vi "Verify Row [  ].vi"(0 "Table size":cluster{"# Column":u16, "# Row":u16}, 7 "Row  [ ] IN":T1) -> (4 "Create Table?":bool, 8 "Row  [ ] OUT":T1)   [LabVIEW 2019]
doc: "Developed by Jean-Marc Simard\nCopyright © 2012, Exaprom Inc.\nAll rights reserved.\nLicense: BSD\n\nWith iTextSharp 4.1.6 (http://itextsharp.sourceforge.net)\nunder Mozilla Public License Version 1.1\n(http://www.mozilla.org/MPL/MPL-1.1.html)"
uses:
  <userlib>/Exaprom PDF/Controls/Table Controls/Table Appearance and Font Row [ ].ctl
  <userlib>/Exaprom PDF/Controls/Table Controls/One Row Appearance.ctl
  <userlib>/Exaprom PDF/Controls/Table Controls/Row from to.ctl
  <userlib>/Exaprom PDF/Controls/Table Controls/Cell, Alignment, LS and Font - hide Vmerge.ctl
  <userlib>/Exaprom PDF/Controls/Table Controls/Cell Type, Alignment and LS.ctl
  <userlib>/Exaprom PDF/Controls/Table Controls/Cell Alignment 20px.ctl
  <userlib>/Exaprom PDF/Controls/Table Controls/Text vertical arrangement.ctl
  <userlib>/Exaprom PDF/Controls/Text Controls/Line spacing.ctl
  <userlib>/Exaprom PDF/Controls/Table Controls/Cell Appearance.ctl
  <userlib>/Exaprom PDF/Controls/Table Controls/Cell Border 20 px.ctl
  <userlib>/Exaprom PDF/Controls/Table Controls/Merge Horizontal.ctl
  <userlib>/Exaprom PDF/Controls/Table Controls/Merge Vertical.ctl
  <userlib>/Exaprom PDF/Controls/Font Controls/Font complete cluster.ctl
  <userlib>/Exaprom PDF/Controls/Font Controls/Font size.ctl
  <userlib>/Exaprom PDF/Controls/Font Controls/Font color.ctl
  <userlib>/Exaprom PDF/Controls/Font Controls/Type and encoding.ctl
  <userlib>/Exaprom PDF/Controls/Text Controls/Unicode/Type and run direction.ctl
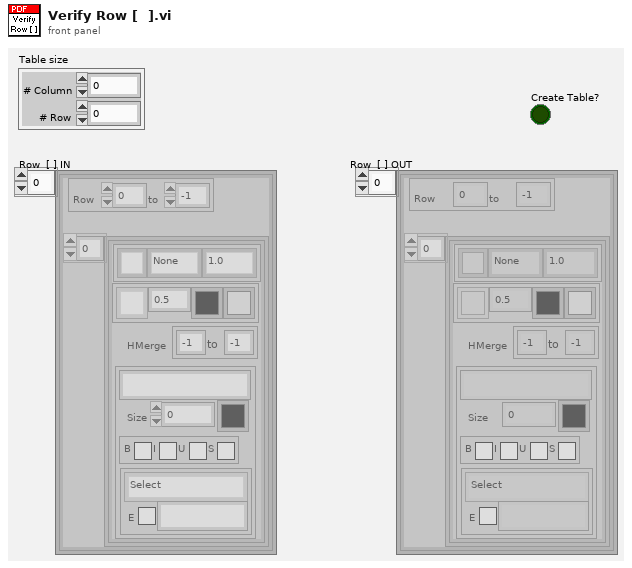
[diagram p1: front panel]
types:
  T1 = typedef "Table Appearance and Font Row [ ].ctl" = T2[]
  T2 = typedef "One Row Appearance.ctl" = cluster{"Row":T3, "Cell [ ]":T4[]}
  T3 = typedef "Row from to.ctl" = cluster{"From #":i16, "to #":i16}
  T4 = typedef "Cell, Alignment, LS and Font - hide Vmerge.ctl" = cluster{"Text":T5, "Cell Appearance":T9, "HMerge":T11, "VMerge":T12, "Font":T13}
  T5 = typedef "Cell Type, Alignment and LS.ctl" = cluster{"Cell Alignment":T6, "Text rotation":T7, "Line spacing":T8}
  T6 = typedef "Cell Alignment 20px.ctl" = u16
  T7 = typedef "Text vertical arrangement.ctl" = enum16{"None", "Clockwise", "Counterclockwise"}
  T8 = typedef "Line spacing.ctl" = enum16{"Select", "1.0", "1.5", "2.0"}
  T9 = typedef "Cell Appearance.ctl" = cluster{"Border":T10, "Thickness":sgl, "Color":u32, "BG":u32}
  T10 = typedef "Cell Border 20 px.ctl" = u16
  T11 = typedef "Merge Horizontal.ctl" = cluster{"From":i8, "to":i8}
  T12 = typedef "Merge Vertical.ctl" = cluster{"From":i8, "to":i8}
  T13 = typedef "Font complete cluster.ctl" = cluster{"Name":string, "Size":T14, "Color":T15, "Style":cluster{"Bold":bool, "Italic":bool, "Underline":bool, "Strikeout":bool}, "Type":T16}
  T14 = typedef "Font size.ctl" = sgl
  T15 = typedef "Font color.ctl" = u32
  T16 = typedef "Type and encoding.ctl" = cluster{"Type&direction":T17, "Embedded":bool, "Encoding":string}
  T17 = typedef "Type and run direction.ctl" = enum16{"Select", "ASCII", "UTF-16", "UTF-16 (default)", "UTF-16 (LTR)", "UTF-16 (RTL)"}
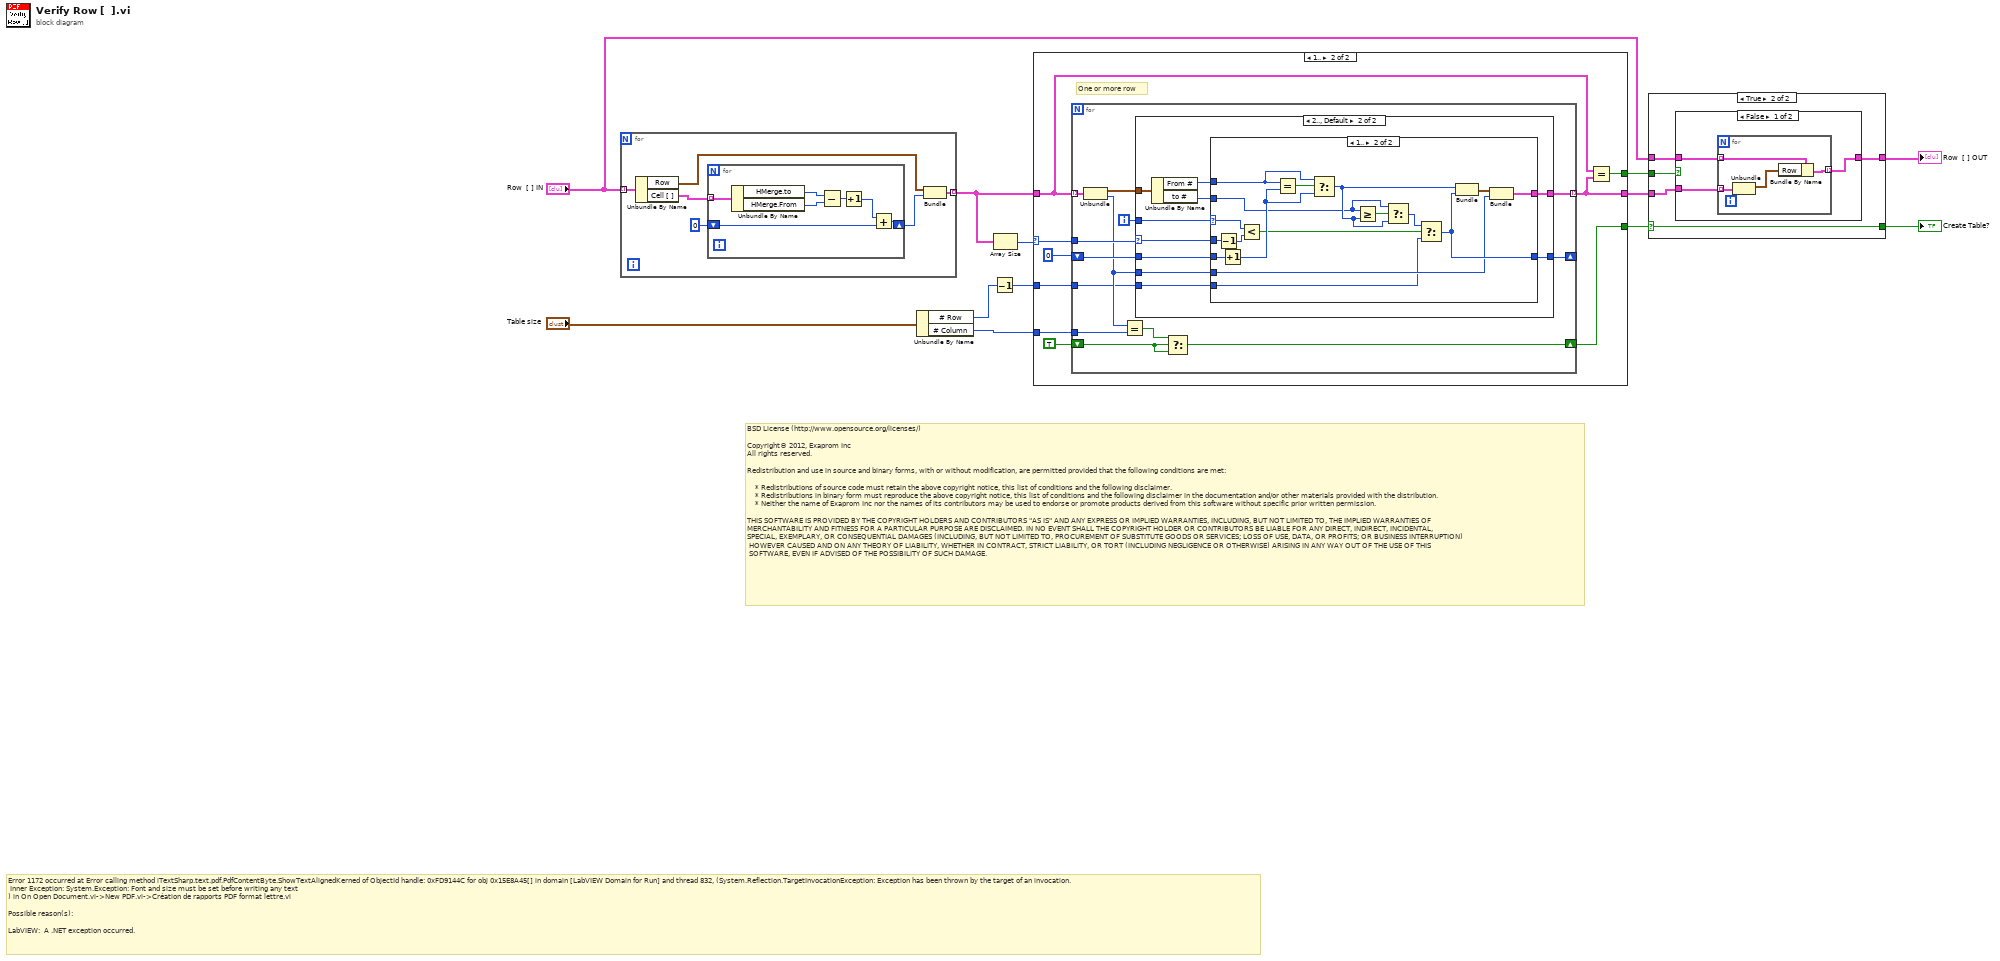
[diagram p0: block diagram]
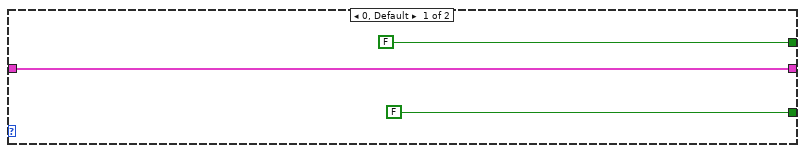
[diagram p4: hidden frame]
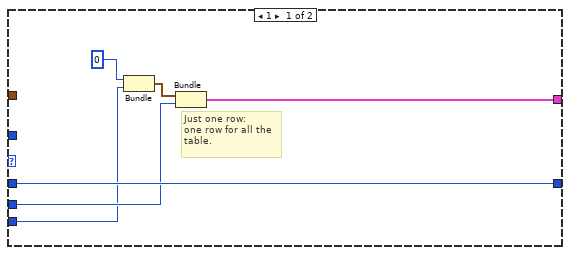
[diagram p5: hidden frame]
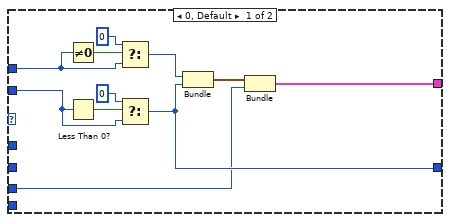
[diagram p6: hidden frame]
diagram:
  # "Error 1172 occurred at Error calling method iTextSharp.text.pdf.PdfContentByte.ShowTextAlignedKerned of ObjectId handle: 0xFD9144C for obj 0x15E8A45[] in domain [LabVIEW Domain for Run] and thread 832, (System.Reflection.TargetInvocationException: Exception has been thrown by the target of an invocation.\n\tInner Exception: System.Exception: Font and size must be set before writing any text\n) in On Open Document.vi->New PDF.vi->Création de rapports PDF format lettre.vi\n\nPossible reason(s):\n\nLabVIEW:  A .NET exception occurred."
  # "BSD License (http://www.opensource.org/licenses/)\n\nCopyright© 2012, Exaprom Inc\nAll rights reserved.\n\nRedistribution and use in source and binary forms, with or without modification, are permitted provided that the following conditions are met:\n\n    * Redistributions of source code must retain the above copyright notice, this list of conditions and the following disclaimer.\n    * Redistributions in binary form must reproduce the above copyright notice, this list of conditions and the following disclaimer in the documentation and/or other materials provided with the distribution.\n    * Neither the name of Exaprom Inc nor the names of its contributors may be used to endorse or promote products derived from this software without specific prior written permission.\n\nTHIS SOFTWARE IS PROVIDED BY THE COPYRIGHT HOLDERS AND CONTRIBUTORS \"AS IS\" AND ANY EXPRESS OR IMPLIED WARRANTIES, INCLUDING, BUT NOT LIMITED TO, THE IMPLIED WARRANTIES OF \nMERCHANTABILITY AND FITNESS FOR A PARTICULAR PURPOSE ARE DISCLAIMED. IN NO EVENT SHALL THE COPYRIGHT HOLDER OR CONTRIBUTORS BE LIABLE FOR ANY DIRECT, INDIRECT, INCIDENTAL,\nSPECIAL, EXEMPLARY, OR CONSEQUENTIAL DAMAGES (INCLUDING, BUT NOT LIMITED TO, PROCUREMENT OF SUBSTITUTE GOODS OR SERVICES; LOSS OF USE, DATA, OR PROFITS; OR BUSINESS INTERRUPTION)\n HOWEVER CAUSED AND ON ANY THEORY OF LIABILITY, WHETHER IN CONTRACT, STRICT LIABILITY, OR TORT (INCLUDING NEGLIGENCE OR OTHERWISE) ARISING IN ANY WAY OUT OF THE USE OF THIS\n SOFTWARE, EVEN IF ADVISED OF THE POSSIBILITY OF SUCH DAMAGE."
  n1 = for {
    tunnel: "Row  [ ] IN" -> [w18] mode=indexing
    tunnel: [w14] -> w12 mode=indexing
    n2 = Unbundle By Name(w18) -> ("Row"=w13:T3, "Cell [ ]"=w17:T4[])
    n3 = for {
      tunnel: w17 -> [w25] mode=indexing
      shift-right: [w20] -> w15
      shift-left: i8 0 -> [w19]
      n4 = Unbundle By Name(w25) -> ("HMerge.to"=w24:i8, "HMerge.From"=w22:i8)
      n5 = Subtract(x=w24, y=w22) -> (x-y=w23:i8)
      n6 = Increment(x=w23) -> (x+1=w21:i8)
      n7 = Add(x=w21, y=w19) -> (x+y=w20:i8)
    }
    n8 = Bundle("Row"=w13, w15) -> (w14:cluster{"Row":T3, i8})  [unwired: 1 in]
  }
  n9 = Unbundle By Name("Table size") -> ("# Row"=w2:u16, "# Column"=w3:u16)
  n10 = Decrement(x=w2) -> (x-1=w1:u16)
  n11 = Array Size(array=w12) -> (size(s)=w11:i32)
  n12 = case shown="1.." w11 {
    selector: w11 -> [_ w37]
    tunnel: w12 -> [w26 w32]
    tunnel: w3 -> [_ w35]
    tunnel: [w26 w33] -> w7
    tunnel: [FALSE w31] -> w9
    tunnel: [FALSE w30] -> w10
    tunnel: w1 -> [_ w29]
    frame 0, Default {
    }
    frame 1.. {
      # "One or more row"
      n13 = for {
        tunnel: w32 -> [w46] mode=indexing
        tunnel: w37 -> [w50]
        shift-right: [w48] -> _
        shift-left: i16 0 ("t") -> [w47]
        tunnel: w35 -> [w43]
        shift-right: [w41] -> w30
        shift-left: TRUE -> [w40]
        tunnel: [w39] -> w33 mode=indexing
        tunnel: w29 -> [w38]
        i -> [w49]
        n14 = Unbundle(w46) -> ("Row"=w45:T3, w44:i8)
        n15 = Equal?(x=w44, y=w43) -> (x = y?=w42:bool)
        n16 = case shown="2.., Default" w50 {
          selector: w50 -> [_ w62]
          tunnel: w49 -> [_ w66]
          tunnel: [w53 w65] -> w39
          tunnel: [w55 w64] -> w48
          tunnel: w47 -> [w55 w63]
          tunnel: w45 -> [_ w59]
          tunnel: w44 -> [w52 w58]
          tunnel: w38 -> [w51 w57]
          frame 1 {
            # "Just one row: \none row for all the\ntable."
            n17 = Bundle("Row.to #"=i16 0, w51) -> (w54:cluster{"Row.to #":i16, u16})  [unwired: 1 in]
            n18 = Bundle(w54, w52) -> (w53:cluster{cluster{"Row.to #":i16, u16}, i8})  [unwired: 1 in]
          }
          frame 2.., Default {
            n19 = Unbundle By Name(w59) -> ("From #"=w61:i16, "to #"=w60:i16)
            n20 = case shown="1.." w66 {
              selector: w66 -> [_ w86]
              tunnel: w61 -> [w76 w91]
              tunnel: w60 -> [w72 w88]
              tunnel: [w69 w80] -> w65
              tunnel: [w70 w82] -> w64
              tunnel: w63 -> [_ w92]
              tunnel: w62 -> [_ w87]
              tunnel: w58 -> [w67 w79]
              tunnel: w57 -> [_ w78]
              frame 0, Default {
                n21 = Not Equal To 0?(x=w76) -> (x != 0?=w77:bool)
                n22 = Less Than 0?(x=w72) -> (x < 0?=w73:bool)
                n23 = Select(t=i16 0, s=w77, f=w76) -> (s? t:f=w71:i16)
                n24 = Select(t=i16 0, s=w73, f=w72) -> (s? t:f=w70:i16)
                n25 = Bundle("From #"=w71, "to #"=w70) -> (w68:cluster{"From #":i16, "to #":i16})  [unwired: 1 in]
                n26 = Bundle(w68, w67) -> (w69:cluster{cluster{"From #":i16, "to #":i16}, i8})  [unwired: 1 in]
              }
              frame 1.. {
                n27 = Decrement(x=w87) -> (x-1=w85:i32)
                n28 = Increment(x=w92) -> (x+1=w90:u16)
                n29 = Less?(x=w86, y=w85) -> (x < y?=w83:bool)
                n30 = Equal?(x=w91, y=w90) -> (x = y?=w94:bool)
                n31 = Select(t=w91, s=w94, f=w90) -> (s? t:f=w89:u16)
                n32 = Greater Or Equal?(x=w88, y=w89) -> (x >= y?=w93:bool)
                n33 = Select(t=w88, s=w93, f=w89) -> (s? t:f=w84:u16)
                n34 = Select(t=w84, s=w83, f=w78) -> (s? t:f=w82:u16)
                n35 = Bundle("From #"=w89, "From #"=w82) -> (w81:cluster{"From #":u16, "From #":u16})  [unwired: 1 in]
                n36 = Bundle(w81, w79) -> (w80:cluster{cluster{"From #":u16, "From #":u16}, i8})  [unwired: 1 in]
              }
            }
          }
        }
        n37 = Select(t=w42, s=w40, f=w40) -> (s? t:f=w41:bool)
      }
      n38 = Equal?(x=w32, y=w33) -> (x = y?=w31:bool)
    }
  }
  n39 = case shown="True" w10 {
    selector: w10 -> [w95 w97]
    tunnel: w9 -> [_ w101]
    tunnel: w7 -> [_ w100]
    tunnel: "Row  [ ] IN" -> [w96 w99]
    tunnel: [w96 w98] -> w6
    tunnel: [w95 w97] -> w5
    frame False {
    }
    frame True {
      n40 = case shown="False" w101 {
        tunnel: w100 -> [w103 _]
        tunnel: w99 -> [w104 w109]
        tunnel: [w102 w109] -> w98
        frame False {
          n41 = for {
            tunnel: w104 -> [w108] mode=indexing
            tunnel: w103 -> [w107] mode=indexing
            tunnel: [w105] -> w102 mode=indexing
            n42 = Unbundle(w107) -> ("Row"=w106:cluster{"From #":u16, "From #":u16})  [unwired: 1 out]
            n43 = Bundle By Name(cluster=w108, "Row"=w106) -> (w105:T2)
          }
        }
        frame True {
        }
      }
    }
  }
  "Row  [ ] OUT" <- w6
  "Create Table?" <- w5
